vi "ReportStartBuild.vi"(0 "Table in":refnum<vi>, 1 "Operator":string, 2 "Numeric in":i32, 3 "GeneralResult-Pass(T)Fail(F)":bool, 4 "Header Array":string[][](array[string]), 5 "error in (no error)":errorcluster, 6 "SN":string) -> (14 "Numeric out":i32, 19 "error out":errorcluster)   [LabVIEW 2017]
uses:
  <vilib>/Utility/sysdir.llb/System Directory Type.ctl
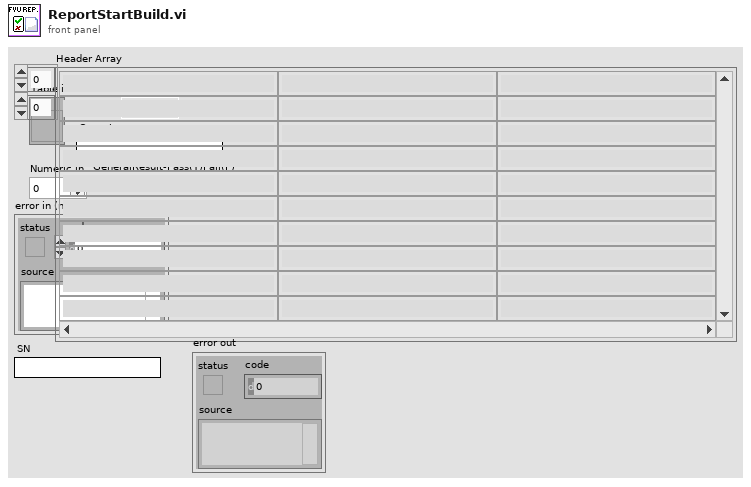
[diagram p1: front panel]
types:
  T1 = typedef "System Directory Type.ctl" = i32
  T2 = enum16{"open", "replace", "create", "open or create", "replace or create", "replace or create with confirmation"}
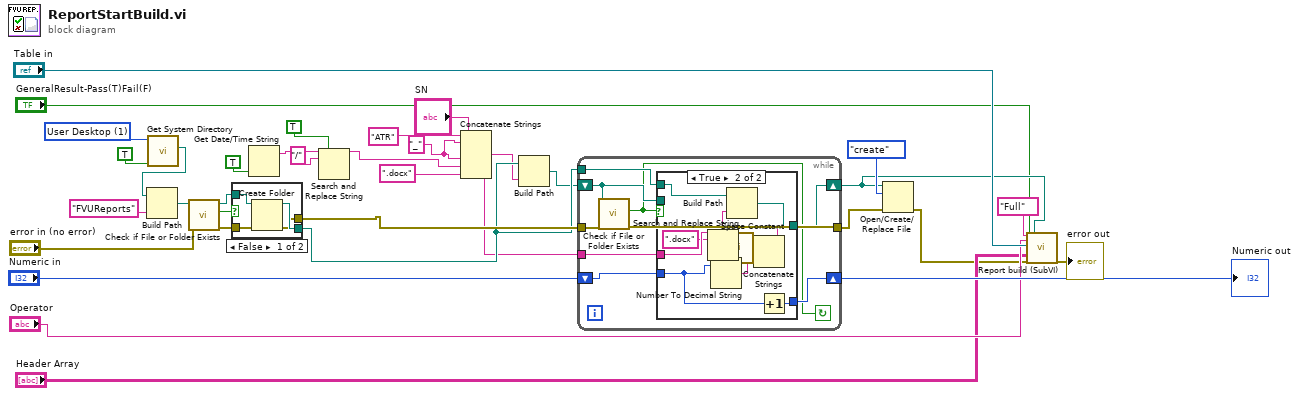
[diagram p0: block diagram]
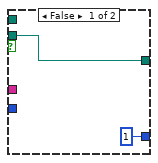
[diagram p2: hidden frame]
diagram:
  w30 = T1 1 items=["User Home"=0, "User Desktop"=1, "User Documents"=2, "User Application Data"=3, "User Preferences"=4, "User Temporary"=5, "Public Documents"=6, "Public Application Data"=7, "Public Preferences"=8, "Public Cache"=13, "System Core Libraries"=9, "System Installed Libraries"=10, "Application Files"=11, "Boot Volume Root"=12] ("system directory type")
  w33 = "_"
  n1 = call <vilib>:"Get System Directory.vi"("create directory if not found? (F)"=TRUE, "system directory type"=w30) -> ("system directory"=w31:path)  [unwired: 9 in]
  n2 = Build Path(base path=w31, name or relative path="FVUReports") -> (appended path=w14:path)
  n3 = call <vilib>:"Check if File or Folder Exists.vi"("error in (no error)"="error in (no error)", "path"=w14) -> ("error out"=w16:errorcluster, "file or folder exists?"=w13:bool, "dup path"=w15:path)  [unwired: 7 in]
  n4 = case shown="False" w13 {
    tunnel: w16 -> [w38 w39]
    tunnel: w15 -> [w37 w40]
    tunnel: [w36 w40] -> w28
    tunnel: [w35 w39] -> w34
    frame False {
      n5 = Create Folder(path (use dialog)=w37, error in=w38) -> (created path=w36:path, error out=w35:errorcluster)  [unwired: 1 in, 1 out]
    }
    frame True {
    }
  }
  n6 = Get Date/Time String(want seconds? (F)=TRUE) -> (date string=w12:string)  [unwired: 2 in, 1 out]
  n7 = Search and Replace String(replace all?=TRUE ("replace all? (F)"), input string=w12, search string="/") -> (result string=w23:string)  [unwired: 5 in, 3 out]
  n8 = Concatenate Strings("ATR" ("string"), w33, "SN", w33, w23, ".docx" ("string")) -> (w25:string)
  n9 = Build Path(base path=w28, name or relative path=w25) -> (appended path=w24:path)
  n10 = while {
    tunnel: w25 -> [w47]
    tunnel: w28 -> [w44]
    shift-right: [w46] -> w6
    shift-left: w24 -> [w45]
    shift-right: [w42] -> w27
    shift-left: "Numeric in" -> [w43]
    tunnel: w34 -> [w48]
    tunnel: [w49] -> w29
    stop <- w41 continue-if-true
    n11 = call <vilib>:"Check if File or Folder Exists.vi"("error in (no error)"=w48, "path"=w45) -> ("error out"=w49:errorcluster, "file or folder exists?"=w41:bool)  [unwired: 7 in, 1 out]
    n12 = case shown="True" w41 {
      tunnel: w47 -> [_ w61]
      tunnel: w43 -> [_ w53]
      tunnel: [w51 w58] -> w46
      tunnel: w45 -> [w51 _]
      tunnel: w44 -> [_ w59]
      tunnel: [1 w52] -> w42
      frame False {
      }
      frame True {
        w54 = ".docx" ("search string")
        n13 = Search and Replace String(input string=w61, search string=w54) -> (result string=w60:string)  [unwired: 6 in, 3 out]
        n14 = Number To Decimal String(number=w53) -> (decimal integer string=w56:string)  [unwired: 1 in]
        n15 = call <vilib>:"Space Constant.vi"() -> ("String"=w55:string)
        n16 = Concatenate Strings(w60, w55, w56, w54) -> (w57:string)
        n17 = Build Path(base path=w59, name or relative path=w57) -> (appended path=w58:path)
        n18 = Increment(x=w53) -> (x+1=w52:i32)
      }
    }
  }
  "Numeric out" <- w27
  n19 = Open/Create/Replace File(file path (use dialog)=w6, error in=w29, operation (0:open)=T2."create") -> (error out=w3:errorcluster)  [unwired: 3 in, 2 out]
  n20 = call "Report build (SubVI).vi"("Full/Fails"="Full", "Operator"="Operator", "Original ATR Ref"="Table in", "GeneralResult-Pass(T)Fail(F)"="GeneralResult-Pass(T)Fail(F)", "Header Array"="Header Array", "error in (no error)"=w3, "report file path"=w6) -> ("error out"=→"error out":errorcluster)  [unwired: 12 in]
